vi "Get Speed.vi"(8 "error in (no error)":errorcluster, 11 "FW102C in":i32) -> (0 "error out":errorcluster, 2 "Speed":enum16{"Slow Speed", "High Speed"}(ring), 3 "FW102C out":i32)   [LabVIEW 2015, in "Thorlabs_FW102C.lvlib"]
doc: "Returns the move profile speed mode"
uses:
  Thorlabs_FW102C.lvlib
  <instrlib>/Thorlabs_FW102C/Library/FilterWheel102_win64.dll
  Library/FilterWheel102_win32.dll
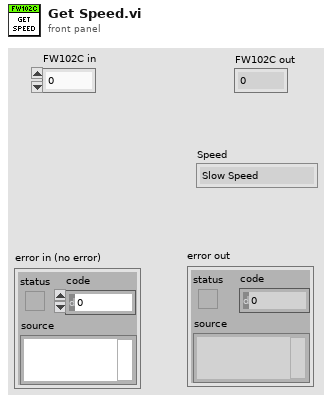
[diagram p1: front panel]
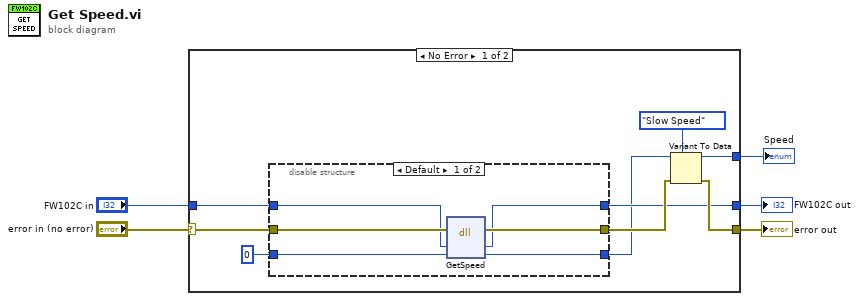
[diagram p0: block diagram]
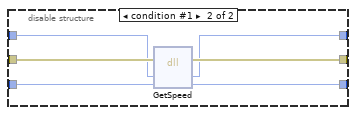
[diagram p2: hidden frame]
diagram:
  n1 = case shown="No Error" "error in (no error)" {
    selector: "error in (no error)" -> [w11 w27]
    tunnel: [w13 w27] -> w5
    tunnel: "FW102C in" -> [w9 w28]
    tunnel: [w8 w28] -> w2
    tunnel: [w14 _] -> w1
    frame No Error {
      n2 = disable-structure shown="Default" {
        disable-tunnel: w11 -> [w20 w26]
        disable-tunnel: [w19 w25] -> w10
        disable-tunnel: w9 -> [w18 w24]
        disable-tunnel: [w17 w23] -> w8
        disable-tunnel: [w16 w22] -> w7
        disable-tunnel: 0 ("speed") -> [w15 w21]
        frame condition #0 (active) {
          n3 = dll-call lib="C:/Users/bspok/Desktop/AppNotes_FW102C_v400/AppNotes_FW102C/LabVIEW/Thorlabs_FW102C/Library/FilterWheel102_win32.dll" fn="GetSpeed"(error in=w20, "hdl"=w18, "speed"=w15) -> (error out=w19:errorcluster, "hdl"=w17:i32, "speed"=w16:i32)  [unwired: 3 in, 1 out]
        }
        frame condition #1 {
          n4 = dll-call lib="D:/Program Files/National Instruments/LabVIEW 2011/instr.lib/Thorlabs_FW102C/Library/FilterWheel102_win64.dll" fn="GetSpeed"(error in=w26, "hdl"=w24, "speed"=w21) -> (error out=w25:errorcluster, "hdl"=w23:i32, "speed"=w22:i32)  [unwired: 3 in, 1 out]
        }
      }
      n5 = Variant To Data(error in=w10, type=enum16{"Slow Speed", "High Speed"}."Slow Speed" ("Speed"), Variant=w7) -> (data=w14:enum16{"Slow Speed", "High Speed"}, error out=w13:errorcluster)
    }
    frame Error {
    }
  }
  "error out" <- w5
  "FW102C out" <- w2
  "Speed" <- w1
